vi "NF LI56xx dvr sTRG.vi"(8 "error in":errorcluster caption="error in (no error)" {"code" format="%.0x"}, 11 "VISA resource name":refnum<visa-resource-name>) -> (0 "error out":errorcluster {"code" format="%.0x"}, 3 "VISA resource name copy":refnum<visa-resource-name>)   [LabVIEW 2019]
doc: "When the measurement data buffer is enabled, executes a trigger and records data in the measurement buffer. \nWhen the internal timer is disabled, measurement data is recorded only once. \nWhen the internal timer is enabled, starts recording measurement data according to the internal timer. \nEnable the measurement data buffer -> :DATA:FEED:CONTrol command\nSet the internal timer -> :DATA:TIMer command\nBefore using triggers, the awaiting trigger state must be set with the :INITiate[:IMMediate] command. An error will result if the awaiting trigger state has not been set."
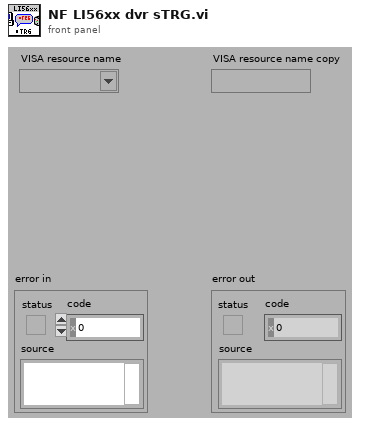
[diagram p1: front panel]
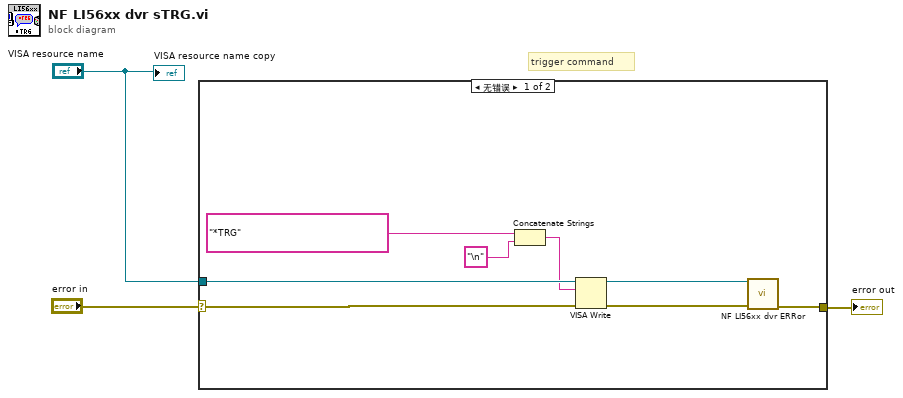
[diagram p0: block diagram]
diagram:
  # "trigger command"
  n1 = case shown="无错误" "error in" {
    selector: "error in" -> [w11 w12]
    tunnel: [w7 w12] -> w3
    tunnel: "VISA resource name" -> [w10 _]
    frame No Error {
      n2 = Concatenate Strings("*TRG" ("•¶Žš—ñ"), "\n" ("Œ`Ž®•¶Žš—ñ")) -> (w5:string)
      n3 = VISA Write(VISA resource name=w10, write buffer=w5, error in (no error)=w11) -> (VISA resource name out=w9:refnum<visa-resource-name>, error out=w8:errorcluster)  [unwired: 1 out]
      n4 = call "NF LI56xx dvr ERRor.vi"("VISA resource name"=w9, "error in (no error)"=w8) -> ("error out"=w7:errorcluster)  [unwired: 10 in, 3 out]
    }
    frame Error {
    }
  }
  "error out" <- w3
  "VISA resource name copy" <- "VISA resource name"
